vi "Add States to Queue Performance Test.vi"() -> ()   [LabVIEW 2013]
panel:
  out "% Improvement":dbl format="%#.1f"
  out "New":u32
  out "Old":u32
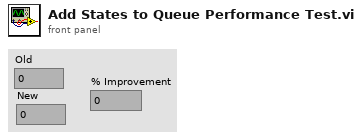
[diagram p1: front panel]
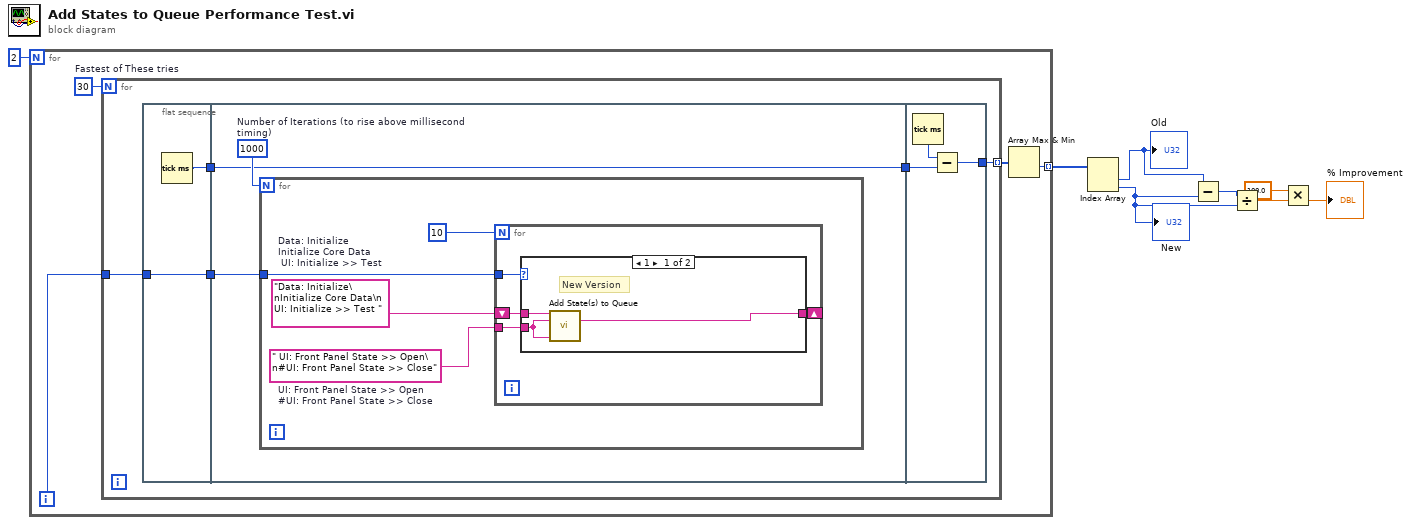
[diagram p0: block diagram]
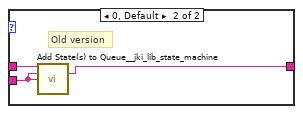
[diagram p2: hidden frame]
diagram:
  n1 = for {
    N: 2 -> [_]
    tunnel: [w9] -> w7 mode=indexing
    i -> [w12]
    w10 = 30  # Fastest of These tries
    n2 = for {
      N: w10 -> [_]
      tunnel: w12 -> [w14]
      tunnel: [w13] -> w11 mode=indexing
      n3 = flat-sequence {
        tunnel: [w19] -> w17
        tunnel: w14 -> [w18]
        tunnel: [w18] -> w16
        tunnel: w17 -> [w21]
        tunnel: [w21] -> w15
        tunnel: w16 -> [w20]
        tunnel: w15 -> [w38]
        tunnel: [w37] -> w13
        frame #0 {
          n4 = Tick Count (ms)() -> (millisecond timer value=w19:u32)
        }
        frame #1 {
          w22 = 1000  # Number of Iterations (to rise above millisecond timing)
          n5 = for {
            N: w22 -> [_]
            tunnel: w20 -> [w25]
            w23 = " UI: Front Panel State >> Open\n#UI: Front Panel State >> Close"  # UI: Front Panel State >> Open #UI: Front Panel State >> Close
            w26 = "Data: Initialize\nInitialize Core Data\n UI: Initialize >> Test "  # Data: Initialize Initialize Core Data  UI: Initialize >> Test
            n6 = for {
              N: 10 ("Numeric") -> [_]
              shift-right: [w29] -> _
              shift-left: w26 -> [w30]
              tunnel: w25 -> [w28]
              tunnel: w23 -> [w27]
              n7 = case shown="1" w28 {
                tunnel: w30 -> [w33 w36]
                tunnel: [w32 w35] -> w29
                tunnel: w27 -> [w31 w34]
                frame 1 {
                  # "New Version"
                  n8 = call "Add State(s) to Queue.vi"("State(s) in Front (\"\")"=w33, "State(s) in (\"\")"=w31, "State(s) at Back (\"\")"=w31) -> ("States Out"=w32:string)  [unwired: 12 in]
                }
                frame 0, Default {
                  # "Old version"
                  n9 = call <vilib>:"Add State(s) to Queue__jki_lib_state_machine.vi"("State(s) in Front (\"\")"=w36, "State(s) in (\"\")"=w34, "State(s) at Back (\"\")"=w34) -> ("States Out"=w35:string)  [unwired: 12 in]
                }
              }
            }
          }
        }
        frame #2 {
          n10 = Tick Count (ms)() -> (millisecond timer value=w39:u32)
          n11 = Subtract(x=w39, y=w38) -> (x-y=w37:u32)
        }
      }
    }
    n12 = Array Max & Min(array=w11) -> (min value=w9:u32)  [unwired: 3 out]
  }
  n13 = Index Array(array=w7) -> (element #1=w5:u32, element #2=w1:u32)  [unwired: 2 in]
  "Old" <- w5
  "New" <- w1
  n14 = Subtract(x=w5, y=w1) -> (x-y=w6:u32)
  n15 = Divide(x=w6, y=w1) -> (x/y=w4:dbl)
  n16 = Multiply(x=100.0, y=w4) -> (x*y=→"% Improvement":dbl)
